vi "Flowmeter conversion.vi"(9 "Required Litres":dbl, 10 "Density Required":dbl) -> (2 "Total Litres (calc)":dbl)   [LabVIEW 2011]
uses:
  Pumps_Valves_Dependencies_Global.vi
panel:
  out "Pulse count":dbl
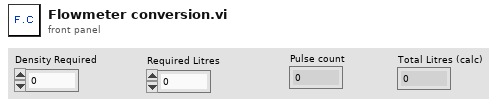
[diagram p1: front panel]
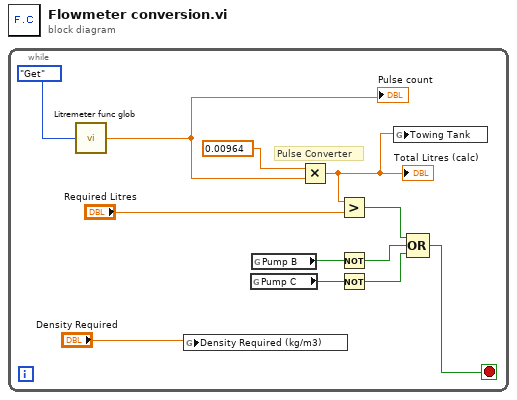
[diagram p0: block diagram]
diagram:
  n1 = while {
    stop <- w2 stop-if-true
    # "Pulse Converter"
    n2 = call "Litremeter func glob.vi"("Action"=enum16{"Get", "Set"}."Get") -> ("Total Litres (calc)"=w11:dbl)  [unwired: 4 in, 4 out]
    "Pulse count" <- w11
    n3 = global write "Pumps_Valves_Dependencies_Global.vi" "Density Required (kg/m3)"("Density Required") -> ()
    n4 = global read "Pumps_Valves_Dependencies_Global.vi" "Pump C"() -> (w7:bool)
    n5 = global read "Pumps_Valves_Dependencies_Global.vi" "Pump B"() -> (w6:bool)
    n6 = Multiply(x=0.00964, y=w11) -> (x*y=w1:dbl)
    "Total Litres (calc)" <- w1
    n7 = Greater?(x=w1, y="Required Litres") -> (0:w5:bool)
    n8 = Not(x=w6) -> (.not. x?=w4:bool)
    n9 = Not(x=w7) -> (.not. x?=w3:bool)
    n10 = global write "Pumps_Valves_Dependencies_Global.vi" "Towing Tank"(w1) -> ()
    n11 = Compound Arithmetic op=OR(w5, w4, w3) -> (w2:bool)
  }
